vi "template-gru-cell_v1.2.vi"(7 "x":T1, 9 "h":T1) -> (1 "h + 1":T1)   [LabVIEW 2020]
uses:
  <vilib>/Analysis/Matrix/Datatypes/RealMatrix.ctl
  <vilib>/Analysis/Matrix/Numeric/Multiply/Multiply - RM,RM.vi
  <vilib>/Analysis/Matrix/Numeric/Add/Add - RM,RM.vi
  <vilib>/Analysis/Matrix/NI_Matrix.lvlib
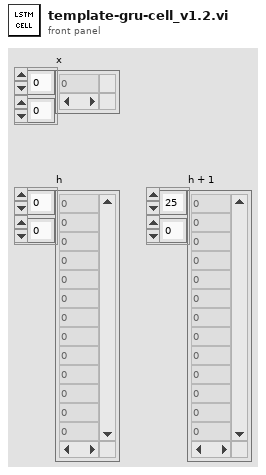
[diagram p1: front panel]
types:
  T1 = typedef "NI_Matrix.lvlib/RealMatrix.ctl" = dbl[][]
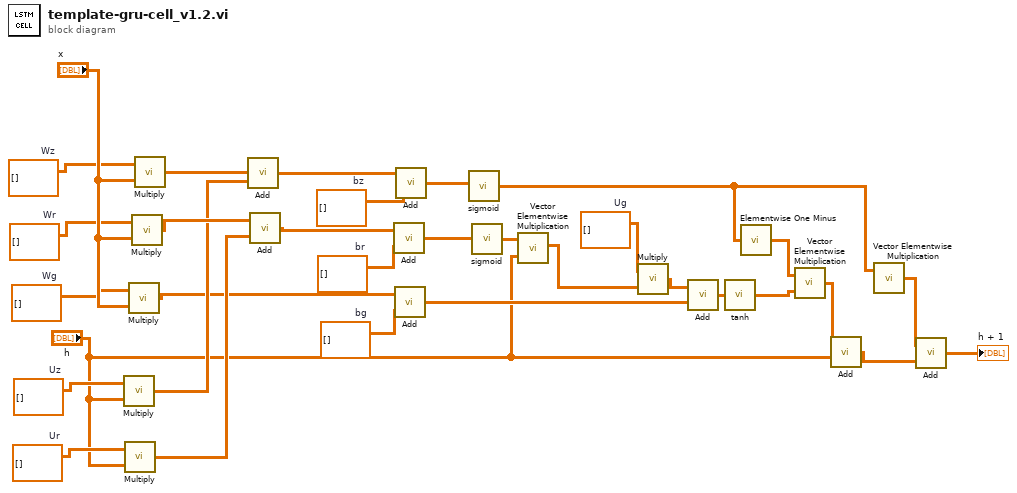
[diagram p0: block diagram]
diagram:
  w13 = T1 []  # Ug
  w18 = T1 []  # bg
  w30 = T1 []  # Wr
  w27 = T1 []  # Ur
  w29 = T1 []  # Wg
  w21 = T1 []  # bz
  w28 = T1 []  # Uz
  w31 = T1 []  # Wz
  w19 = T1 []  # br
  n1 = call-poly <vilib>:"Multiply.vi"("Real Matrix B"="h", "Real Matrix A"=w28) -> ("A * B"=w24:T1)
  n2 = call-poly <vilib>:"Multiply.vi"("Real Matrix B"="h", "Real Matrix A"=w27) -> ("A * B"=w23:T1)
  n3 = call-poly <vilib>:"Multiply.vi"("Real Matrix B"="x", "Real Matrix A"=w29) -> ("A * B"=w14:T1)
  n4 = call-poly <vilib>:"Multiply.vi"("Real Matrix B"="x", "Real Matrix A"=w30) -> ("A * B"=w25:T1)
  n5 = call-poly <vilib>:"Multiply.vi"("Real Matrix B"="x", "Real Matrix A"=w31) -> ("A * B"=w26:T1)
  n6 = call-poly <vilib>:"Add.vi"("Real Matrix B"=w24, "Real Matrix A"=w26) -> ("A + B"=w22:T1)
  n7 = call-poly <vilib>:"Add.vi"("Real Matrix B"=w23, "Real Matrix A"=w25) -> ("A + B"=w20:T1)
  n8 = call-poly <vilib>:"Add.vi"("Real Matrix B"=w19, "Real Matrix A"=w20) -> ("A + B"=w16:T1)
  n9 = call-poly <vilib>:"Add.vi"("Real Matrix B"=w18, "Real Matrix A"=w14) -> ("A + B"=w10:T1)
  n10 = call-poly <vilib>:"Add.vi"("Real Matrix B"=w21, "Real Matrix A"=w22) -> ("A + B"=w17:T1)
  n11 = call "sigmoid.vi"("x"=w17) -> ("y"=w8:T1)
  n12 = call "sigmoid.vi"("x"=w16) -> ("y"=w15:T1)
  n13 = call "Vector Elementwise Multiplication.vi"("Matrix 1"="h", "Matrix in"=w15) -> ("elementwise product"=w12:T1)
  n14 = call-poly <vilib>:"Multiply.vi"("Real Matrix B"=w12, "Real Matrix A"=w13) -> ("A * B"=w11:T1)
  n15 = call-poly <vilib>:"Add.vi"("Real Matrix B"=w10, "Real Matrix A"=w11) -> ("A + B"=w9:T1)
  n16 = call "tanh.vi"("x"=w9) -> ("y"=w6:T1)
  n17 = call "Elementwise One Minus.vi"("x"=w8) -> ("y"=w7:T1)
  n18 = call "Vector Elementwise Multiplication.vi"("Matrix 1"=w6, "Matrix in"=w7) -> ("elementwise product"=w5:T1)
  n19 = call-poly <vilib>:"Add.vi"("Real Matrix B"="h", "Real Matrix A"=w5) -> ("A + B"=w3:T1)
  n20 = call "Vector Elementwise Multiplication.vi"("Matrix in"=w8) -> ("elementwise product"=w2:T1)  [unwired: 1 in]
  n21 = call-poly <vilib>:"Add.vi"("Real Matrix B"=w3, "Real Matrix A"=w2) -> ("A + B"=→"h + 1":T1)
